vi "read binary file or zipped binary file.vi"(8 "error in":errorcluster, 11 "File":path) -> (0 "error out":errorcluster, 3 "data":string)   [LabVIEW 2018]
uses:
  <vilib>/zip/NI_Unzip.lvlib
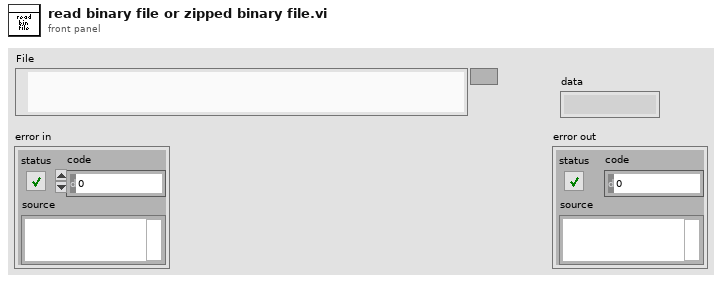
[diagram p1: front panel]
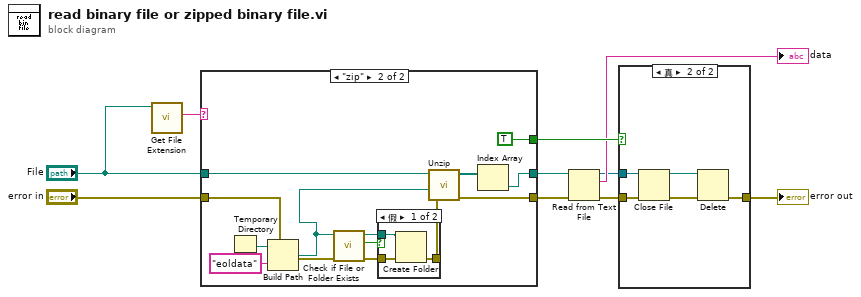
[diagram p0: block diagram]
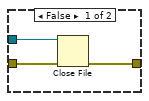
[diagram p2: hidden frame]
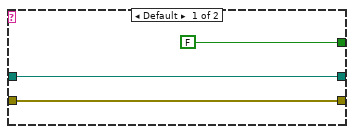
[diagram p3: hidden frame]
diagram:
  n1 = call <vilib>:"Get File Extension.vi"("file"="File") -> ("lowercase file extension"=w3:string)  [unwired: 6 in, 4 out]
  n2 = case shown="\"zip\"" w3 {
    tunnel: [w13 w23] -> w4
    tunnel: "File" -> [w13 w26]
    tunnel: "error in" -> [w12 w18]
    tunnel: [w12 w25] -> w7
    tunnel: [FALSE TRUE] -> w8
    frame Default {
    }
    frame "zip" {
      n3 = Temporary Directory() -> (w21:path)
      n4 = Build Path(base path=w21, name or relative path="eoldata") -> (appended path=w19:path)
      n5 = call <vilib>:"Check if File or Folder Exists.vi"("error in (no error)"=w18, "path"=w19) -> ("error out"=w16:errorcluster, "file or folder exists?"=w17:bool, "dup path"=w14:path)  [unwired: 7 in]
      n6 = case shown="假" w17 {
        tunnel: w16 -> [w29 w30]
        tunnel: [w27 w30] -> w15
        tunnel: w14 -> [w28 _]
        frame False {
          n7 = Create Folder(path (use dialog)=w28, error in=w29) -> (error out=w27:errorcluster)  [unwired: 1 in, 2 out]
        }
        frame True {
        }
      }
      n8 = call <vilib>:"Unzip.vi"("error in (no error)"=w15, "Target directory (same as Zip file if empty)"=w19, "Zip file"=w26) -> ("error out"=w25:errorcluster, "Unzipped files"=w24:path[])  [unwired: 6 in, 1 out]
      n9 = Index Array(array=w24) -> (element=w23:path)  [unwired: 1 in]
    }
  }
  n10 = Read from Text File(file (use dialog)=w4, error in=w7) -> (refnum out=w1:refnum<file>, text=→"data":string, error out=w9:errorcluster)  [unwired: 2 in, 1 out]
  n11 = case shown="真" w8 {
    tunnel: w9 -> [w32 w37]
    tunnel: [w31 w38] -> w10
    tunnel: w1 -> [w33 w35]
    frame False {
      n12 = Close File(refnum=w33, error in=w32) -> (error out=w31:errorcluster)  [unwired: 1 out]
    }
    frame True {
      n13 = Close File(refnum=w35, error in=w37) -> (path=w34:path, error out=w36:errorcluster)
      n14 = Delete(path (use dialog)=w34, error in=w36) -> (error out=w38:errorcluster)  [unwired: 3 in, 2 out]
    }
  }
  "error out" <- w10
